vi "Periodic Tasks.vi"(8 "error in (no error)":errorcluster) -> ()   [LabVIEW 2012]
doc: "This VI runs in parallel to other tasks. It can contain as many user-defined periodic loops as you need. These can carry out PID or other sorts of timed response."
uses:
  <vilib>/Rock Robotics/SystemInterfaces/Utilities/FPGA_UtilitiesLED Source.ctl
  <vilib>/Rock Robotics/SystemInterfaces/Utilities/FPGA_UtilitiesLED State.ctl
  Robot Global Data.vi
  <vilib>/Rock Robotics/WPI/RobotDrive/WPI_RobotDriveGetSetRefNum.vi
  <vilib>/Rock Robotics/WPI/RobotDrive/WPI_RobotDriveArcadeDrive_Standard(NoSaturation).vi
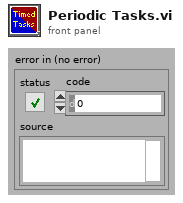
[diagram p1: front panel]
types:
  T1 = typedef "WPI_CompressorDevRef.ctl" = cluster{"DevStatus":errorcluster, "DigitalInputDevRef":T2, "RelayDevRef":T5}
  T2 = typedef "WPI_DigitalInputDevRef.ctl" = cluster{"DevStatus":errorcluster, "DIO Channel":T3, "Digital Module":T4}
  T3 = typedef "FPGA_DIOChannel.ctl" = enum8{"DIO 1", "DIO 2", "DIO 3", "DIO 4", "DIO 5", "DIO 6", "DIO 7", "DIO 8", "DIO 9", "DIO 10", "DIO 11", "DIO 12", "DIO 13", "DIO 14", "Invalid"}
  T4 = typedef "FPGA_TypedefDigitalModule.ctl" = enum16{"Digital Module 1", "Digital Module 2"}
  T5 = typedef "WPI_RelayDevRef.ctl" = cluster{"DevStatus":errorcluster, "Relay Channel":T6, "Digital Module":T4, "Relay Direction":T7}
  T6 = typedef "FPGA_DIORelayChannel.ctl" = enum8{"Relay 1", "Relay 2", "Relay 3", "Relay 4", "Relay 5", "Relay 6", "Relay 7", "Relay 8", "Invalid"}
  T7 = typedef "WPI_RelayDirection.ctl" = enum16{"Both directions", "Forward only", "Reverse only"}
  T8 = typedef "FPGA_UtilitiesLED State.ctl" = enum16{"Off", "On", "Toggle"}
  T9 = typedef "FPGA_UtilitiesLED Source.ctl" = enum16{"User LED", "FPGA LED"}
  T10 = typedef "WPI_MotorControlDeviceRef.ctl" = cluster{"DeviceStatus":errorcluster, "Type":enum16{"PWM", "CAN"}, "PWM":cluster{"Digital Module":T4, "PWM Channel":T11, "DeadBand":T12}, "CAN":cluster{"Device Number":u8, "Control Mode":T13, "Semaphore":T14, "Max Vout":dbl}, "Invert":bool, "TransformRef":T15, "InvTransformRef":T15}
  T11 = typedef "FPGA_DIOPWMChannel.ctl" = enum8{"PWM 1", "PWM 2", "PWM 3", "PWM 4", "PWM 5", "PWM 6", "PWM 7", "PWM 8", "PWM 9", "PWM 10", "Invalid"}
  T12 = typedef "WPI_PWMDeadband.ctl" = cluster{"Name":string, "maxPositivePwm":i32, "minPositivePwm":i32, "centerPwm":i32, "maxNegativePwm":i32, "minNegativePwm":i32, "angularRange":u16}
  T13 = typedef "WPI_CANJaguar_ControlMode.ctl" = enum8{"Percent VBus", "Current", "Speed", "Position", "Voltage"}
  T14 = typedef "Semaphore RefNum" = refnum<k1>
  T15 = typedef "WPI_PWMTransform_ConPane.ctl" = refnum<vi>
  T16 = typedef "WPI_EncoderDevRef.ctl" = cluster{"DevStatus":errorcluster, "EncoderIndex":T17, "CounterIndex":T18, "DistancePerCount":dbl, "Decoding Type":T19}
  T17 = typedef "FPGA_EncoderIdx.ctl" = enum8{"Enc 0", "Enc 1", "Enc 2", "Enc 3", "Invalid"}
  T18 = typedef "FPGA_CounterCtrSystemIndex.ctl" = enum8{"Ctr 0", "Ctr 1", "Ctr 2", "Ctr 3", "Ctr 4", "Ctr 5", "Ctr 6", "Ctr 7", "Invalid"}
  T19 = typedef "WPI_EncoderType.ctl" = enum16{"1x", "2x", "4x"}
  T20 = typedef "WPI_UltrasonicDeviceRef.ctl" = cluster{"DevStatus":errorcluster, "Ping Digital Module":T4, "Echo Digital Module":T4, "Ping Channel":T3, "Echo Channel":T3, "CntIndex":T18}
  T21 = typedef "WPI_RobotDriveDevRef.ctl" = cluster{"DevStatus":errorcluster, "Motors[]":T10[], "Square Inputs":bool, "Max Output":dbl, "Isochronous":bool}
  T22 = typedef "WPI_DigitalOutputDevRef.ctl" = cluster{"Digital Module":T4, "DIO Channel":T3, "DevStatus":errorcluster}
  T23 = typedef "WPI_CounterDevRef.ctl" = cluster{"DevStatus":errorcluster, "CntIndex":T18}
  T24 = typedef "WPI_DriverStationRobotMode2.ctl" = enum16{"Autonomous Disabled", "Autonomous Enabled", "Teleop Disabled", "Teleop Enabled", "Timeout", "Finish", "Test Disabled", "Test Enabled"}
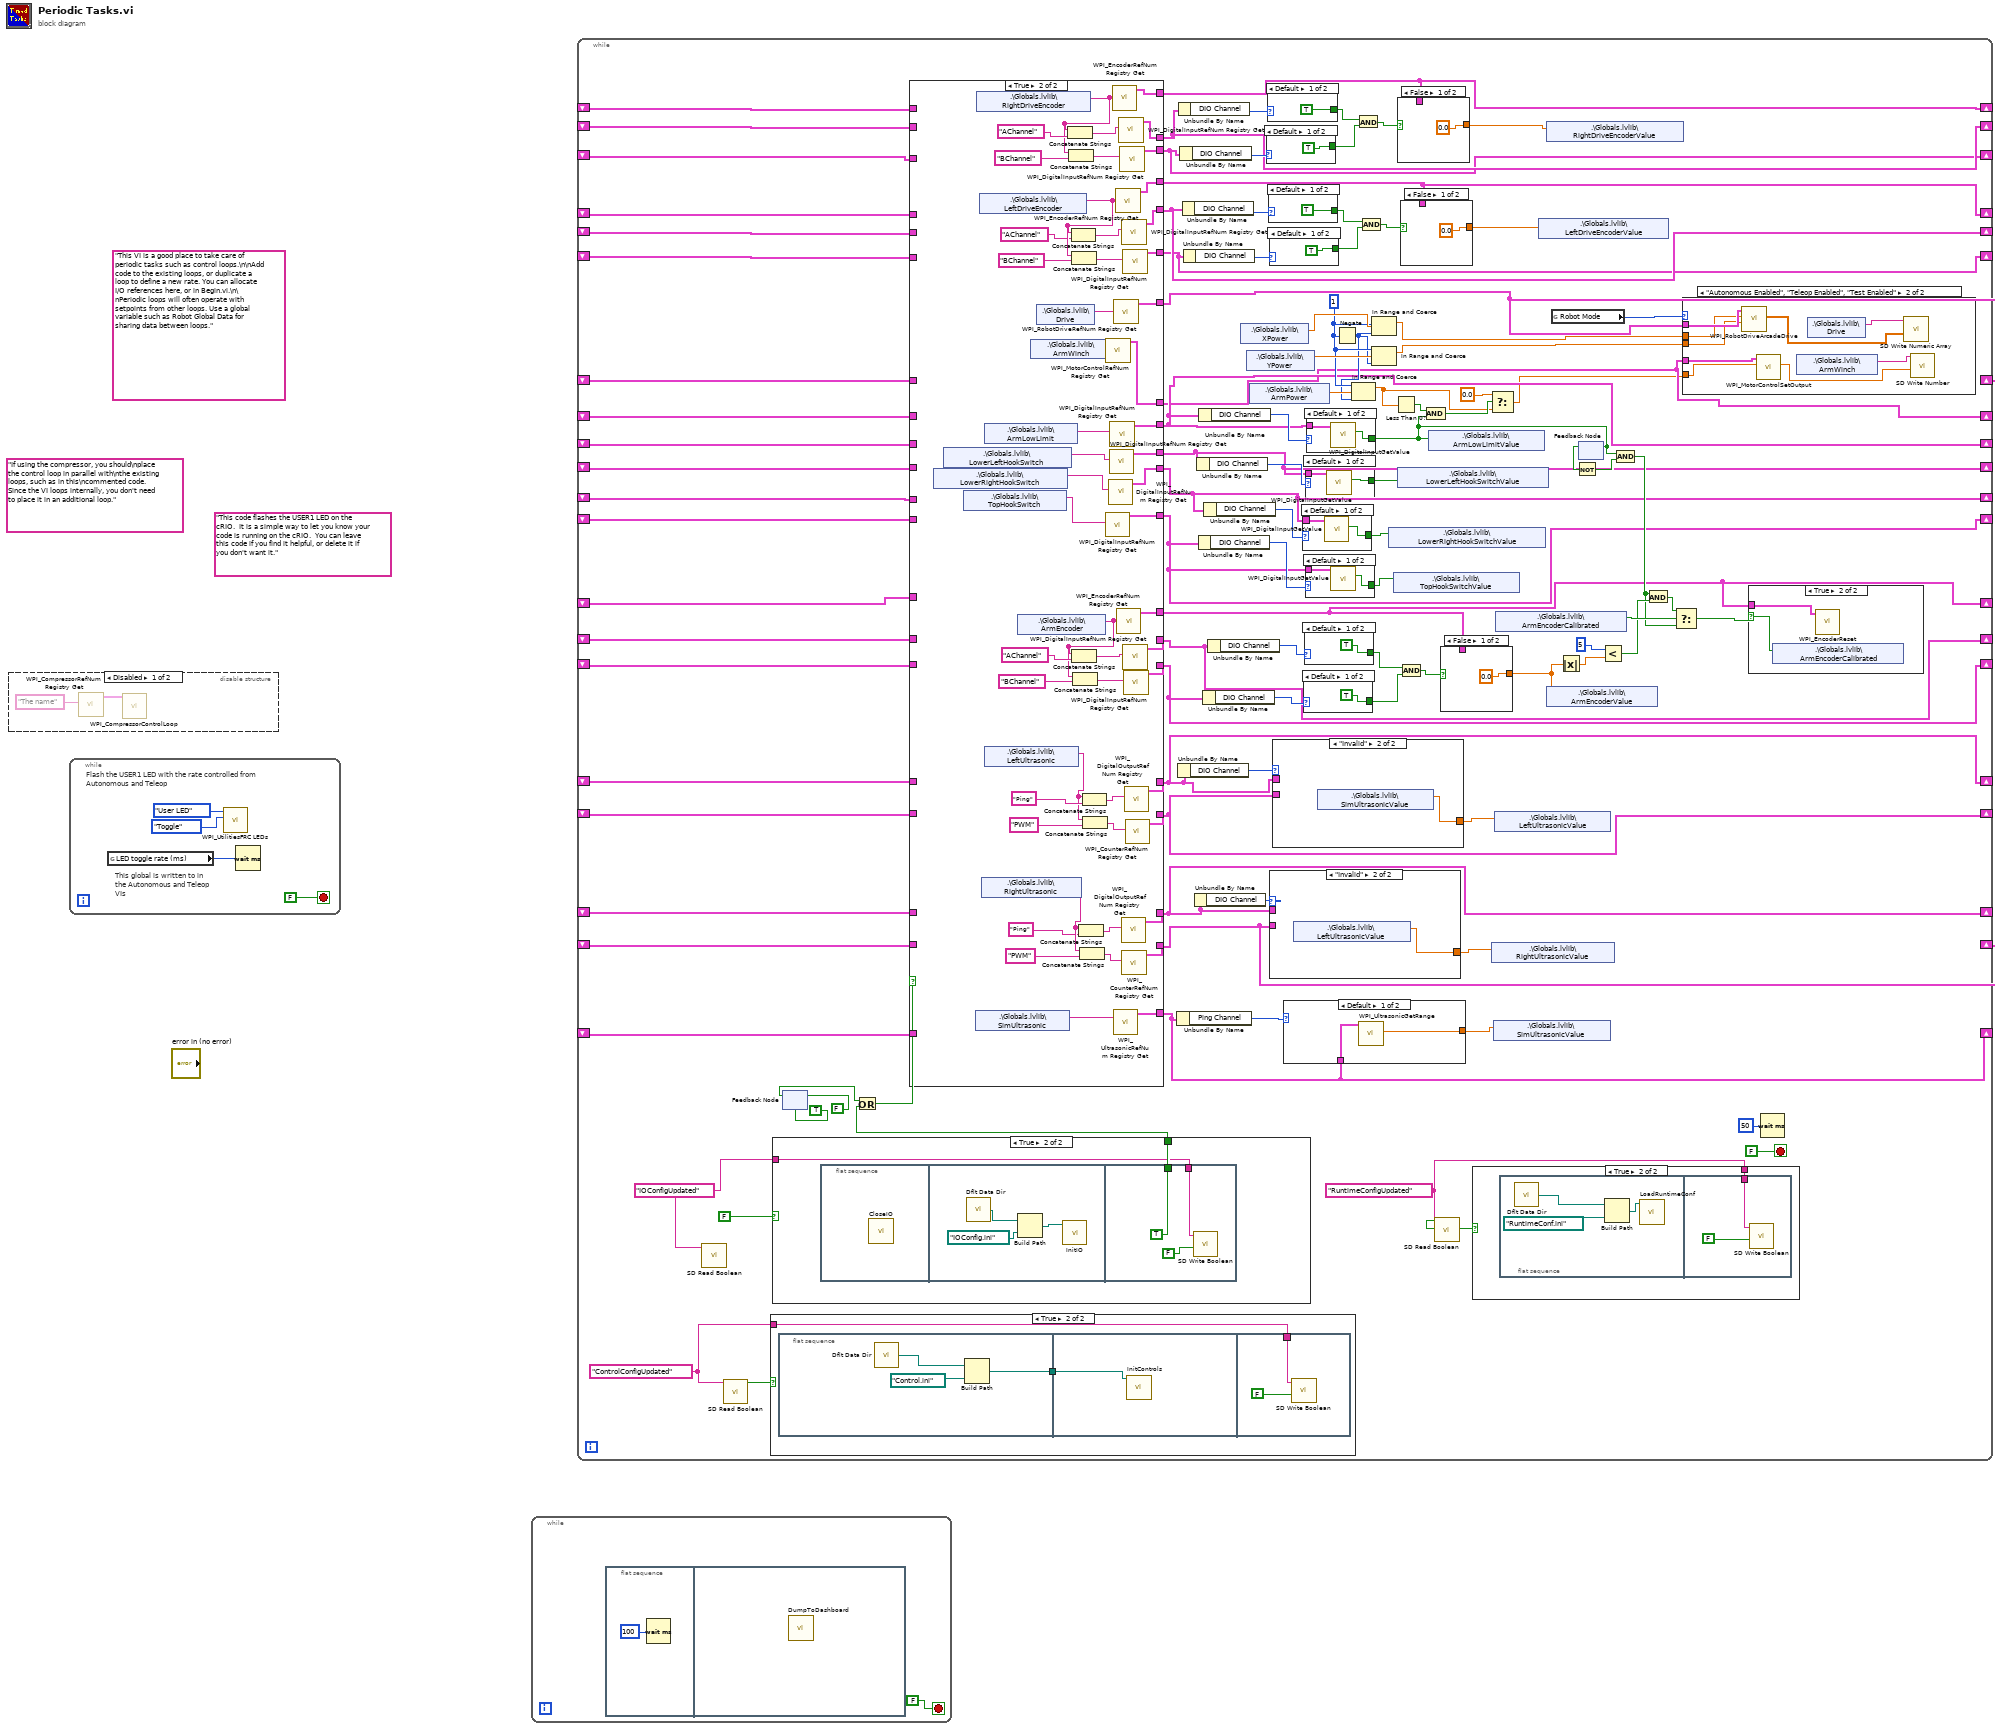
[diagram p0: block diagram]
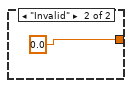
[diagram p3: hidden frame]
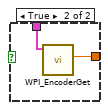
[diagram p5: hidden frame]
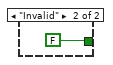
[diagram p6: hidden frame]
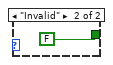
[diagram p7: hidden frame]
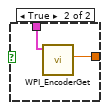
[diagram p8: hidden frame]
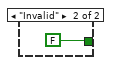
[diagram p9: hidden frame]
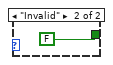
[diagram p10: hidden frame]
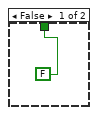
[diagram p12: hidden frame]
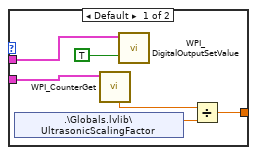
[diagram p16: hidden frame]
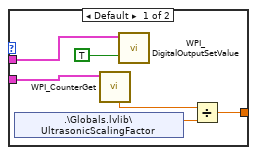
[diagram p17: hidden frame]
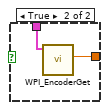
[diagram p18: hidden frame]
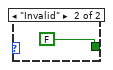
[diagram p19: hidden frame]
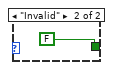
[diagram p20: hidden frame]
diagram:
  (unwired) "If using the compressor, you should\nplace the control loop in parallel with\nthe existing loops, such as in this\ncommented code. Since the VI loops internally, you don't need to place it in an additional loop."
  (unwired) "This code flashes the USER1 LED on the cRIO.  It is a simple way to let you know your code is running on the cRIO.  You can leave this code if you find it helpful, or delete it if you don't want it."
  (unwired) "This VI is a good place to take care of periodic tasks such as control loops.\n\nAdd code to the existing loops, or duplicate a loop to define a new rate. You can allocate I/O references here, or in Begin.vi.\n\nPeriodic loops will often operate with setpoints from other loops. Use a global variable such as Robot Global Data for sharing data between loops."
  n1 = disable-structure shown="Disabled" {
    frame Disabled {
      n2 = call <vilib>:"WPI_CompressorRefNum Registry Get.vi"("refnum name"="The name") -> ("CompressorDevRef"=w2:T1)  [unwired: 9 in, 1 out]
      n3 = call <vilib>:"WPI_CompressorControlLoop.vi"("CompressorDevRef"=w2) -> ()  [unwired: 11 in]
    }
    frame Enabled {
    }
  }
  n4 = while {
    stop <- FALSE stop-if-true
    # "This global is written to in the Autonomous and Teleop VIs"
    # "Flash the USER1 LED with the rate controlled from Autonomous and Teleop"
    n5 = global read "Robot Global Data.vi" "LED toggle rate (ms)"() -> (w3:u32)
    n6 = call <vilib>:"WPI_UtilitiesFRC LEDs.vi"("State"=FPGA_UtilitiesLED_State."Toggle", "LED Type"=FPGA_UtilitiesLED_Source."User LED") -> ()  [unwired: 1 in, 9 out]
    n7 = Wait (ms)(milliseconds to wait=w3) -> ()  [unwired: 1 out]
  }
  n8 = while {
    stop <- FALSE stop-if-true
    n9 = flat-sequence {
      frame #0 {
        n10 = Wait (ms)(milliseconds to wait=u32 100) -> ()  [unwired: 1 out]
      }
      frame #1 {
        n11 = call "DumpToDashboard.vi"() -> ()  [unwired: 12 in]
      }
    }
  }
  n12 = while {
    shift-right: [w17] -> _
    shift-left: _ -> [w75]
    shift-right: [w14] -> _
    shift-left: _ -> [w74]
    shift-right: [w63] -> _
    shift-left: _ -> [w73]
    shift-right: [w62] -> _
    shift-left: _ -> [w72]
    shift-right: [w61] -> _
    shift-left: _ -> [w71]
    shift-right: [w60] -> _
    shift-left: _ -> [w70]
    shift-right: [w58] -> _
    shift-left: _ -> [w69]
    shift-right: [w59] -> _
    shift-left: _ -> [w68]
    shift-right: [w57] -> _
    shift-left: _ -> [w67]
    shift-right: [w56] -> _
    shift-left: _ -> [w64]
    shift-right: [w55] -> _
    shift-left: _ -> [w65]
    shift-right: [w54] -> _
    shift-left: _ -> [w66]
    shift-right: [w53] -> _
    shift-left: _ -> [w52]
    shift-right: [w30] -> _
    shift-left: _ -> [w36]
    shift-right: [w29] -> _
    shift-left: _ -> [w35]
    shift-right: [w28] -> _
    shift-left: _ -> [w33]
    shift-right: [w27] -> _
    shift-left: _ -> [w34]
    shift-right: [w26] -> _
    shift-left: _ -> [w32]
    shift-right: [w25] -> _
    shift-left: _ -> [w31]
    shift-right: [w9] -> _
    shift-left: _ -> [w12]
    stop <- FALSE stop-if-true
    w49 = "RuntimeConfigUpdated"
    w51 = "IOConfigUpdated"
    w76 = "ControlConfigUpdated"
    w91 = 1
    n13 = call <vilib>:"SD Read Boolean.vi"("Name"=w51) -> ()  [unwired: 8 in, 3 out]
    n14 = call <vilib>:"SD Read Boolean.vi"("Name"=w76) -> ("Boolean"=w77:bool)  [unwired: 8 in, 2 out]
    n15 = case shown="True" w77 {
      tunnel: w76 -> [_ w229]
      frame False {
      }
      frame True {
        n16 = flat-sequence {
          tunnel: [w232] -> w230
          tunnel: w230 -> [w234]
          tunnel: w229 -> [w236]
          frame #0 {
            n17 = call <vilib>:"Dflt Data Dir.vi"() -> ("App:Default Data Directory"=w231:path)
            n18 = Build Path(base path=w231, name or relative path=path "Control.ini") -> (appended path=w232:path)
          }
          frame #1 {
            n19 = call "InitControls.vi"("Config"=w234) -> ()  [unwired: 11 in]
          }
          frame #2 {
            n20 = call <vilib>:"SD Write Boolean.vi"("Boolean"=FALSE, "Name"=w236) -> ()  [unwired: 8 in, 2 out]
          }
        }
      }
    }
    n21 = case shown="True" FALSE {
      tunnel: [FALSE w150] -> w23
      tunnel: w51 -> [_ w149]
      frame False {
      }
      frame True {
        n22 = flat-sequence {
          tunnel: [TRUE] -> w150
          tunnel: w149 -> [w154]
          frame #0 {
            n23 = call "CloseIO.vi"() -> ()  [unwired: 12 in]
          }
          frame #1 {
            n24 = call <vilib>:"Dflt Data Dir.vi"() -> ("App:Default Data Directory"=w152:path)
            n25 = Build Path(base path=w152, name or relative path=path "IOConfig.ini") -> (appended path=w151:path)
            n26 = call "InitIO.vi"("Path"=w151) -> ()  [unwired: 11 in]
          }
          frame #2 {
            n27 = call <vilib>:"SD Write Boolean.vi"("Boolean"=FALSE, "Name"=w154) -> ()  [unwired: 8 in, 2 out]
          }
        }
      }
    }
    n28 = feedback-in #1(FALSE) -> ()
    n29 = feedback #1(TRUE) -> (w20:bool)
    n30 = Or(x=w20, y=w23) -> (x .or. y?=w22:bool)
    n31 = case shown="True" w22 {
      tunnel: [w175 w226] -> w14
      tunnel: [w176 w225] -> w17
      tunnel: [w174 w220] -> w63
      tunnel: [w172 w219] -> w61
      tunnel: [w173 w218] -> w62
      tunnel: [w170 w217] -> w60
      tunnel: [w169 w211] -> w59
      tunnel: [w168 w210] -> w58
      tunnel: [w166 w204] -> w56
      tunnel: [w167 w203] -> w57
      tunnel: [w165 w202] -> w55
      tunnel: [w164 w201] -> w54
      tunnel: w75 -> [w176 _]
      tunnel: w74 -> [w175 _]
      tunnel: w73 -> [w174 _]
      tunnel: w72 -> [w173 _]
      tunnel: w71 -> [w172 _]
      tunnel: w70 -> [w170 _]
      tunnel: w69 -> [w168 _]
      tunnel: w68 -> [w169 _]
      tunnel: w67 -> [w167 _]
      tunnel: w66 -> [w164 _]
      tunnel: w65 -> [w165 _]
      tunnel: w64 -> [w166 _]
      tunnel: [w171 w195] -> w53
      tunnel: w52 -> [w171 _]
      tunnel: [w158 w189] -> w25
      tunnel: [w159 w188] -> w26
      tunnel: [w160 w187] -> w27
      tunnel: [w161 w186] -> w28
      tunnel: [w162 w179] -> w29
      tunnel: [w163 w180] -> w30
      tunnel: w36 -> [w163 _]
      tunnel: w35 -> [w162 _]
      tunnel: w34 -> [w160 _]
      tunnel: w33 -> [w161 _]
      tunnel: w32 -> [w159 _]
      tunnel: w31 -> [w158 _]
      tunnel: [w157 w177] -> w9
      tunnel: w12 -> [w157 _]
      frame False {
      }
      frame True {
        n32 = shared-variable ".\\Globals.lvlib\\LowerRightHookSwitch"() -> (w223:string)  [unwired: 1 in, 1 out]
        n33 = shared-variable ".\\Globals.lvlib\\LowerLeftHookSwitch"() -> (w222:string)  [unwired: 1 in, 1 out]
        n34 = shared-variable ".\\Globals.lvlib\\TopHookSwitch"() -> (w224:string)  [unwired: 1 in, 1 out]
        n35 = shared-variable ".\\Globals.lvlib\\SimUltrasonic"() -> (w178:string)  [unwired: 1 in, 1 out]
        n36 = shared-variable ".\\Globals.lvlib\\RightDriveEncoder"() -> (w184:string)  [unwired: 1 in, 1 out]
        n37 = shared-variable ".\\Globals.lvlib\\LeftDriveEncoder"() -> (w191:string)  [unwired: 1 in, 1 out]
        n38 = shared-variable ".\\Globals.lvlib\\RightUltrasonic"() -> (w198:string)  [unwired: 1 in, 1 out]
        n39 = shared-variable ".\\Globals.lvlib\\ArmLowLimit"() -> (w221:string)  [unwired: 1 in, 1 out]
        n40 = shared-variable ".\\Globals.lvlib\\LeftUltrasonic"() -> (w207:string)  [unwired: 1 in, 1 out]
        n41 = shared-variable ".\\Globals.lvlib\\ArmEncoder"() -> (w215:string)  [unwired: 1 in, 1 out]
        n42 = shared-variable ".\\Globals.lvlib\\ArmWinch"() -> (w227:string)  [unwired: 1 in, 1 out]
        n43 = shared-variable ".\\Globals.lvlib\\Drive"() -> (w228:string)  [unwired: 1 in, 1 out]
        n44 = Concatenate Strings(w184, "AChannel") -> (w181:string)
        n45 = Concatenate Strings(w184, "BChannel") -> (w182:string)
        n46 = Concatenate Strings(w191, "AChannel") -> (w194:string)
        n47 = Concatenate Strings(w191, "BChannel") -> (w193:string)
        n48 = Concatenate Strings(w215, "AChannel") -> (w212:string)
        n49 = Concatenate Strings(w215, "BChannel") -> (w213:string)
        n50 = Concatenate Strings(w198, "Ping") -> (w199:string)
        n51 = Concatenate Strings(w198, "PWM") -> (w200:string)
        n52 = Concatenate Strings(w207, "Ping") -> (w206:string)
        n53 = Concatenate Strings(w207, "PWM") -> (w205:string)
        n54 = call <vilib>:"WPI_DigitalInputRefNum Registry Get.vi"("refnum name"=w224) -> ("DigitalInputDevRef"=w195:T2)  [unwired: 9 in, 1 out]
        n55 = call <vilib>:"WPI_MotorControlRefNum Registry Get.vi"("refnum name"=w227) -> ("MotorControlDevRef"=w226:T10)  [unwired: 9 in, 1 out]
        n56 = call <vilib>:"WPI_DigitalInputRefNum Registry Get.vi"("refnum name"=w223) -> ("DigitalInputDevRef"=w219:T2)  [unwired: 9 in, 1 out]
        n57 = call <vilib>:"WPI_DigitalInputRefNum Registry Get.vi"("refnum name"=w222) -> ("DigitalInputDevRef"=w218:T2)  [unwired: 9 in, 1 out]
        n58 = call <vilib>:"WPI_DigitalInputRefNum Registry Get.vi"("refnum name"=w221) -> ("DigitalInputDevRef"=w220:T2)  [unwired: 9 in, 1 out]
        n59 = call <vilib>:"WPI_EncoderRefNum Registry Get.vi"("refnum name"=w184) -> ("EncoderDevRef"=w180:T16)  [unwired: 9 in, 1 out]
        n60 = call <vilib>:"WPI_UltrasonicRefNum Registry Get.vi"("refnum name"=w178) -> ("UltrasonicDevRef"=w177:T20)  [unwired: 9 in, 1 out]
        n61 = call <vilib>:"WPI_RobotDriveRefNum Registry Get.vi"("refnum name"=w228) -> ("RobotDriveDevRef"=w225:T21)  [unwired: 9 in, 1 out]
        n62 = call <vilib>:"WPI_EncoderRefNum Registry Get.vi"("refnum name"=w191) -> ("EncoderDevRef"=w187:T16)  [unwired: 9 in, 1 out]
        n63 = call <vilib>:"WPI_EncoderRefNum Registry Get.vi"("refnum name"=w215) -> ("EncoderDevRef"=w217:T16)  [unwired: 9 in, 1 out]
        n64 = call <vilib>:"WPI_DigitalInputRefNum Registry Get.vi"("refnum name"=w181) -> ("DigitalInputDevRef"=w179:T2)  [unwired: 9 in, 1 out]
        n65 = call <vilib>:"WPI_DigitalInputRefNum Registry Get.vi"("refnum name"=w182) -> ("DigitalInputDevRef"=w186:T2)  [unwired: 9 in, 1 out]
        n66 = call <vilib>:"WPI_DigitalOutputRefNum Registry Get.vi"("refnum name"=w199) -> ("DigitalOutputDevRef"=w202:T22)  [unwired: 9 in, 1 out]
        n67 = call <vilib>:"WPI_DigitalInputRefNum Registry Get.vi"("refnum name"=w194) -> ("DigitalInputDevRef"=w188:T2)  [unwired: 9 in, 1 out]
        n68 = call <vilib>:"WPI_CounterRefNum Registry Get.vi"("refnum name"=w200) -> ("CounterDevRef"=w201:T23)  [unwired: 9 in, 1 out]
        n69 = call <vilib>:"WPI_DigitalInputRefNum Registry Get.vi"("refnum name"=w193) -> ("DigitalInputDevRef"=w189:T2)  [unwired: 9 in, 1 out]
        n70 = call <vilib>:"WPI_DigitalInputRefNum Registry Get.vi"("refnum name"=w212) -> ("DigitalInputDevRef"=w211:T2)  [unwired: 9 in, 1 out]
        n71 = call <vilib>:"WPI_DigitalInputRefNum Registry Get.vi"("refnum name"=w213) -> ("DigitalInputDevRef"=w210:T2)  [unwired: 9 in, 1 out]
        n72 = call <vilib>:"WPI_DigitalOutputRefNum Registry Get.vi"("refnum name"=w206) -> ("DigitalOutputDevRef"=w203:T22)  [unwired: 9 in, 1 out]
        n73 = call <vilib>:"WPI_CounterRefNum Registry Get.vi"("refnum name"=w205) -> ("CounterDevRef"=w204:T23)  [unwired: 9 in, 1 out]
      }
    }
    n74 = Unbundle By Name(w9) -> ("Ping Channel"=w11:T3)
    n75 = Unbundle By Name(w57) -> ("DIO Channel"=w98:T3)
    n76 = Unbundle By Name(w29) -> ("DIO Channel"=w40:T3)
    n77 = Unbundle By Name(w28) -> ("DIO Channel"=w39:T3)
    n78 = Unbundle By Name(w26) -> ("DIO Channel"=w47:T3)
    n79 = Unbundle By Name(w25) -> ("DIO Channel"=w48:T3)
    n80 = Unbundle By Name(w55) -> ("DIO Channel"=w95:T3)
    n81 = Unbundle By Name(w62) -> ("DIO Channel"=w109:T3)
    n82 = Unbundle By Name(w53) -> ("DIO Channel"=w107:T3)
    n83 = Unbundle By Name(w63) -> ("DIO Channel"=w110:T3)
    n84 = Unbundle By Name(w58) -> ("DIO Channel"=w102:T3)
    n85 = Unbundle By Name(w61) -> ("DIO Channel"=w108:T3)
    n86 = Unbundle By Name(w59) -> ("DIO Channel"=w103:T3)
    n87 = shared-variable ".\\Globals.lvlib\\XPower"() -> (w94:dbl)  [unwired: 1 in, 1 out]
    n88 = shared-variable ".\\Globals.lvlib\\YPower"() -> (w93:dbl)  [unwired: 1 in, 1 out]
    n89 = shared-variable ".\\Globals.lvlib\\ArmPower"() -> (w90:dbl)  [unwired: 1 in, 1 out]
    n90 = case shown="Default" w39 {
      tunnel: [TRUE FALSE] -> w43
      frame Default {
      }
      frame "Invalid" {
      }
    }
    n91 = case shown="Default" w40 {
      tunnel: [TRUE FALSE] -> w42
      frame Default {
      }
      frame "Invalid" {
      }
    }
    n92 = case shown="Default" w47 {
      tunnel: [TRUE FALSE] -> w45
      frame Default {
      }
      frame "Invalid" {
      }
    }
    n93 = case shown="Default" w48 {
      tunnel: [TRUE FALSE] -> w44
      frame Default {
      }
      frame "Invalid" {
      }
    }
    n94 = case shown="\"Invalid\"" w95 {
      tunnel: w55 -> [w243 _]
      tunnel: w54 -> [w244 _]
      tunnel: [w239 w245] -> w96
      frame Default {
        n95 = shared-variable ".\\Globals.lvlib\\UltrasonicScalingFactor"() -> (w241:dbl)  [unwired: 1 in, 1 out]
        n96 = call <vilib>:"WPI_CounterGet.vi"("CounterDevRef in"=w244) -> ("Period (sec)"=w240:dbl)  [unwired: 5 in, 5 out]
        n97 = call <vilib>:"WPI_DigitalOutputSetValue.vi"("Value"=TRUE, "DigitalOutputDevRef"=w243) -> ()  [unwired: 8 in, 2 out]
        n98 = Divide(x=w240, y=w241) -> (x/y=w239:dbl)
      }
      frame "Invalid" {
        n99 = shared-variable ".\\Globals.lvlib\\LeftUltrasonicValue"() -> (w245:dbl)  [unwired: 1 in, 1 out]
      }
    }
    n100 = case shown="\"Invalid\"" w98 {
      tunnel: w57 -> [w250 _]
      tunnel: w56 -> [w251 _]
      tunnel: [w246 w252] -> w97
      frame Default {
        n101 = shared-variable ".\\Globals.lvlib\\UltrasonicScalingFactor"() -> (w248:dbl)  [unwired: 1 in, 1 out]
        n102 = call <vilib>:"WPI_CounterGet.vi"("CounterDevRef in"=w251) -> ("Period (sec)"=w247:dbl)  [unwired: 5 in, 5 out]
        n103 = call <vilib>:"WPI_DigitalOutputSetValue.vi"("Value"=TRUE, "DigitalOutputDevRef"=w250) -> ()  [unwired: 8 in, 2 out]
        n104 = Divide(x=w247, y=w248) -> (x/y=w246:dbl)
      }
      frame "Invalid" {
        n105 = shared-variable ".\\Globals.lvlib\\SimUltrasonicValue"() -> (w252:dbl)  [unwired: 1 in, 1 out]
      }
    }
    n106 = case shown="Default" w11 {
      tunnel: [w116 0.0] -> w10
      tunnel: w9 -> [w117 _]
      frame Default {
        n107 = call <vilib>:"WPI_UltrasonicGetRange.vi"("UltrasonicDevRef"=w117) -> ("Distance"=w116:dbl)  [unwired: 8 in, 2 out]
      }
      frame "Invalid" {
      }
    }
    n108 = case shown="Default" w108 {
      tunnel: [w264 FALSE] -> w105
      tunnel: w61 -> [w263 _]
      frame Default {
        n109 = call <vilib>:"WPI_DigitalInputGetValue.vi"("DigitalInputDevRef"=w263) -> ("Value"=w264:bool)  [unwired: 8 in, 2 out]
      }
      frame "Invalid" {
      }
    }
    n110 = case shown="Default" w102 {
      tunnel: [TRUE FALSE] -> w100
      frame Default {
      }
      frame "Invalid" {
      }
    }
    n111 = case shown="Default" w103 {
      tunnel: [TRUE FALSE] -> w101
      frame Default {
      }
      frame "Invalid" {
      }
    }
    n112 = case shown="Default" w109 {
      tunnel: [w267 FALSE] -> w104
      tunnel: w62 -> [w266 _]
      frame Default {
        n113 = call <vilib>:"WPI_DigitalInputGetValue.vi"("DigitalInputDevRef"=w266) -> ("Value"=w267:bool)  [unwired: 8 in, 2 out]
      }
      frame "Invalid" {
      }
    }
    n114 = case shown="Default" w107 {
      tunnel: [w261 FALSE] -> w106
      tunnel: w53 -> [w260 _]
      frame Default {
        n115 = call <vilib>:"WPI_DigitalInputGetValue.vi"("DigitalInputDevRef"=w260) -> ("Value"=w261:bool)  [unwired: 8 in, 2 out]
      }
      frame "Invalid" {
      }
    }
    n116 = case shown="Default" w110 {
      tunnel: [w270 FALSE] -> w80
      tunnel: w63 -> [w269 _]
      frame Default {
        n117 = call <vilib>:"WPI_DigitalInputGetValue.vi"("DigitalInputDevRef"=w269) -> ("Value"=w270:bool)  [unwired: 8 in, 2 out]
      }
      frame "Invalid" {
      }
    }
    n118 = Negate(x=w91) -> (-x=w89:i32)
    n119 = In Range and Coerce(upper limit=w91, x=w90, lower limit=w89) -> (coerced(x)=w92:dbl)  [unwired: 1 out]
    n120 = And(x=w42, y=w43) -> (x .and. y?=w41:bool)
    n121 = And(x=w45, y=w44) -> (x .and. y?=w46:bool)
    n122 = In Range and Coerce(upper limit=w91, x=w94, lower limit=w89) -> (coerced(x)=w16:dbl)  [unwired: 1 out]
    n123 = In Range and Coerce(upper limit=w91, x=w93, lower limit=w89) -> (coerced(x)=w15:dbl)  [unwired: 1 out]
    n124 = shared-variable ".\\Globals.lvlib\\LowerRightHookSwitchValue"(w105) -> ()  [unwired: 1 in, 1 out]
    n125 = shared-variable ".\\Globals.lvlib\\TopHookSwitchValue"(w106) -> ()  [unwired: 1 in, 1 out]
    n126 = Less Than 0?(x=w92) -> (x < 0?=w113:bool)
    n127 = case shown="False" w41 {
      tunnel: w30 -> [_ w130]
      tunnel: [0.0 w129] -> w37
      frame False {
      }
      frame True {
        n128 = call <vilib>:"WPI_EncoderGet.vi"("EncoderDevRef"=w130) -> ("Distance"=w129:dbl)  [unwired: 5 in, 5 out]
      }
    }
    n129 = shared-variable ".\\Globals.lvlib\\LowerLeftHookSwitchValue"(w104) -> ()  [unwired: 1 in, 1 out]
    n130 = And(x=w101, y=w100) -> (x .and. y?=w99:bool)
    n131 = case shown="False" w46 {
      tunnel: w27 -> [_ w137]
      tunnel: [0.0 w136] -> w38
      frame False {
      }
      frame True {
        n132 = call <vilib>:"WPI_EncoderGet.vi"("EncoderDevRef"=w137) -> ("Distance"=w136:dbl)  [unwired: 5 in, 5 out]
      }
    }
    n133 = And(x=w113, y=w80) -> (x .and. y?=w112:bool)
    n134 = shared-variable ".\\Globals.lvlib\\ArmLowLimitValue"(w80) -> ()  [unwired: 1 in, 1 out]
    n135 = call <vilib>:"SD Read Boolean.vi"("Name"=w49) -> ("Boolean"=w50:bool)  [unwired: 8 in, 2 out]
    n136 = case shown="False" w99 {
      tunnel: w60 -> [_ w255]
      tunnel: [0.0 w254] -> w88
      frame False {
      }
      frame True {
        n137 = call <vilib>:"WPI_EncoderGet.vi"("EncoderDevRef"=w255) -> ("Distance"=w254:dbl)  [unwired: 5 in, 5 out]
      }
    }
    n138 = case shown="True" w50 {
      tunnel: w49 -> [_ w142]
      frame False {
      }
      frame True {
        n139 = flat-sequence {
          tunnel: w142 -> [w147]
          frame #0 {
            n140 = call <vilib>:"Dflt Data Dir.vi"() -> ("App:Default Data Directory"=w145:path)
            n141 = Build Path(base path=w145, name or relative path=path "RuntimeConf.ini") -> (appended path=w143:path)
            n142 = call "LoadRuntimeConf.vi"("Path"=w143) -> ()  [unwired: 11 in]
          }
          frame #1 {
            n143 = call <vilib>:"SD Write Boolean.vi"("Boolean"=FALSE, "Name"=w147) -> ()  [unwired: 8 in, 2 out]
          }
        }
      }
    }
    n144 = Select(t=0.0, s=w112, f=w92) -> (s? t:f=w13:dbl)
    n145 = shared-variable ".\\Globals.lvlib\\RightUltrasonicValue"(w96) -> ()  [unwired: 1 in, 1 out]
    n146 = shared-variable ".\\Globals.lvlib\\SimUltrasonicValue"(w10) -> ()  [unwired: 1 in, 1 out]
    n147 = shared-variable ".\\Globals.lvlib\\LeftUltrasonicValue"(w97) -> ()  [unwired: 1 in, 1 out]
    n148 = shared-variable ".\\Globals.lvlib\\ArmEncoderCalibrated"() -> (w85:bool)  [unwired: 1 in, 1 out]
    n149 = shared-variable ".\\Globals.lvlib\\LeftDriveEncoderValue"(w38) -> ()  [unwired: 1 in, 1 out]
    n150 = shared-variable ".\\Globals.lvlib\\RightDriveEncoderValue"(w37) -> ()  [unwired: 1 in, 1 out]
    n151 = shared-variable ".\\Globals.lvlib\\ArmEncoderValue"(w88) -> ()  [unwired: 1 in, 1 out]
    n152 = global read "Robot Global Data.vi" "Robot Mode"() -> (w18:T24)
    n153 = Absolute Value(x=w88) -> (abs(x)=w87:dbl)
    n154 = feedback #2() -> (w81:bool)  [unwired: 1 in]
    n155 = Not(x=w81) -> (.not. x?=w79:bool)
    n156 = feedback-in #2(w80) -> ()
    n157 = Less?(x=5, y=w87) -> (x < y?=w84:bool)
    n158 = And(x=w80, y=w79) -> (x .and. y?=w78:bool)
    n159 = And(x=w78, y=w84) -> (x .and. y?=w83:bool)
    n160 = Select(t=w83, s=w85, f=w78) -> (s? t:f=w82:bool)
    n161 = case shown="\"Autonomous Enabled\", \"Teleop Enabled\", \"Test Enabled\"" w18 {
      tunnel: w17 -> [_ w127]
      tunnel: w16 -> [_ w126]
      tunnel: w15 -> [_ w125]
      tunnel: w14 -> [_ w124]
      tunnel: w13 -> [_ w123]
      frame Default {
      }
      frame "Autonomous Enabled", "Teleop Enabled", "Test Enabled" {
        n162 = call-poly <vilib>:"WPI_RobotDriveArcadeDrive.vi"("Y axis value"=w125, "X axis value"=w126, "RobotDriveDevRef"=w127) -> ("Motor Values"=w119:dbl[])  [unwired: 6 in, 2 out]
        n163 = call <vilib>:"WPI_MotorControlSetOutput.vi"("Output"=w123, "MotorControlDevRef"=w124) -> ("Motor Output"=w122:dbl)  [unwired: 7 in, 2 out]
        n164 = shared-variable ".\\Globals.lvlib\\ArmWinch"() -> (w121:string)  [unwired: 1 in, 1 out]
        n165 = shared-variable ".\\Globals.lvlib\\Drive"() -> (w120:string)  [unwired: 1 in, 1 out]
        n166 = call <vilib>:"SD Write Numeric Array.vi"("Numeric Array"=w119, "Name"=w120) -> ()  [unwired: 8 in, 2 out]
        n167 = call <vilib>:"SD Write Number.vi"("Numeric"=w122, "Name"=w121) -> ()  [unwired: 8 in, 2 out]
      }
    }
    n168 = case shown="True" w82 {
      selector: w82 -> [_ w237]
      tunnel: w60 -> [_ w238]
      frame False {
      }
      frame True {
        n169 = shared-variable ".\\Globals.lvlib\\ArmEncoderCalibrated"(w237) -> ()  [unwired: 1 in, 1 out]
        n170 = call <vilib>:"WPI_EncoderReset.vi"("EncoderDevRef"=w238) -> ()  [unwired: 9 in, 2 out]
      }
    }
    n171 = Wait (ms)(milliseconds to wait=u32 50) -> ()  [unwired: 1 out]
  }
